vi "generuj_eventy.vi"(10 "lambda":dbl=1.0, 11 "Godziny":i32) -> (3 "Array":T1[](array[typedef]))   [LabVIEW 2013]
doc: "Losuje tablicę eventów (przybyć klientów), klienci przychodzą przez \"Godziny\" godzin. Losowanie jest zgodne z procesem Poissona z parametrem \"lambda\"."
uses:
  event.ctl
  ModelowanieLABVIEW_copy/LukiBrary.lvlib
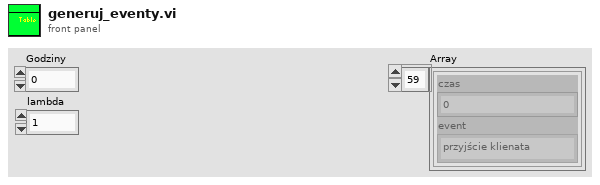
[diagram p1: front panel]
types:
  T1 = typedef "event.ctl" = cluster{"czas":u32, "event":enum16{"przyjście klienata", "zwolnienie kasy", "oczekiwanie na klienta", "nowy event"}}
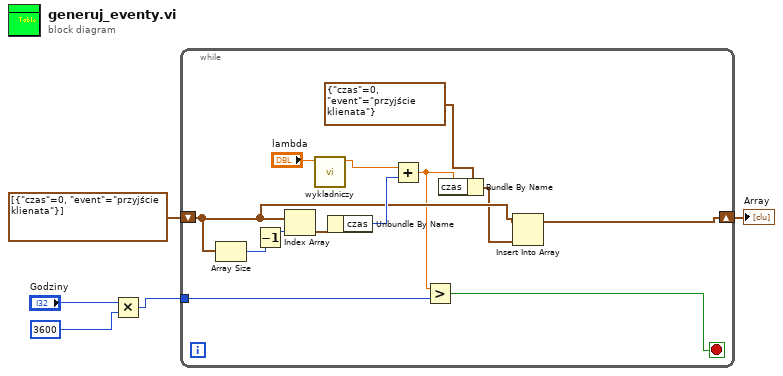
[diagram p0: block diagram]
diagram:
  n1 = Multiply(x="Godziny", y=3600) -> (x*y=w2:i32)
  n2 = while {
    shift-right: [w9] -> w1
    shift-left: T1[] [{"czas"=0, "event"=enum."przyjście klienata"}] -> [w11]
    tunnel: w2 -> [w8]
    stop <- w6 stop-if-true
    n3 = Array Size(array=w11) -> (size(s)=w17:i32)
    n4 = Decrement(x=w17) -> (x-1=w16:i32)
    n5 = Index Array(array=w11, index=w16) -> (element=w15:T1)
    n6 = call "wykladniczy.vi"("lambda"="lambda") -> ("X~wykładniczy"=w13:dbl)  [unwired: 10 in]
    n7 = Unbundle By Name(w15) -> ("czas"=w12:u32)
    n8 = Add(x=w13, y=w12) -> (x+y=w7:dbl)
    n9 = Greater?(x=w7, y=w8) -> (0:w6:bool)
    n10 = Bundle By Name(cluster=T1 {"czas"=0, "event"=enum."przyjście klienata"} ("Cluster"), "czas"=w7) -> (w10:T1)
    n11 = Insert Into Array(array=w11, new element=w10) -> (w9:T1[])  [unwired: 1 in]
  }
  "Array" <- w1
